vi "Terminate Session.vi"(8 "error in (no error)":errorcluster, 10 "Destroy (T)":bool=TRUE, 11 "Session in":refnum<class "Session.lvclass">) -> (0 "error out":errorcluster, 2 "Destroyed":bool, 3 "Session out":refnum<class "Session.lvclass">)   [LabVIEW 2013, in "MQTT Server.lvlib" / "Session.lvclass"]
doc: "Set the \"Destroy\" flag to True if the Connection Handler terminates to force the session to be destroyed for good, no matter what the CleanSession flag state is.\nIf the Connection Handler does not terminate and the CleanSession flag is false, then the Session's process stops but the last state of the session is maintained for a possible client reconnection."
uses:
  Session.lvclass
  Session.lvclass/Session.ctl
  Connection/TCPConnection.lvclass
  StoredSessions/StoredSessions.lvclass
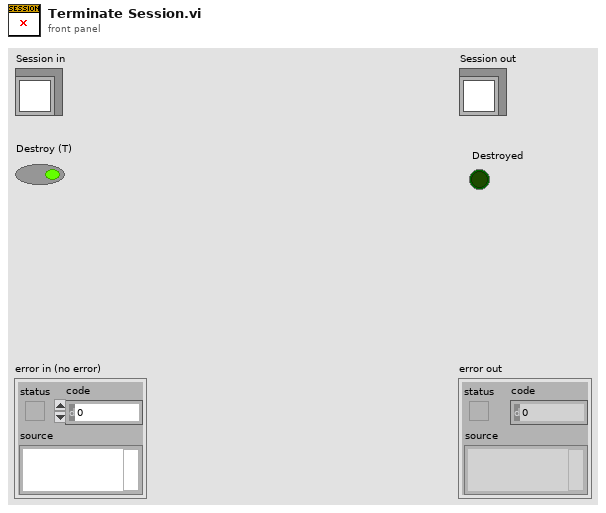
[diagram p1: front panel]
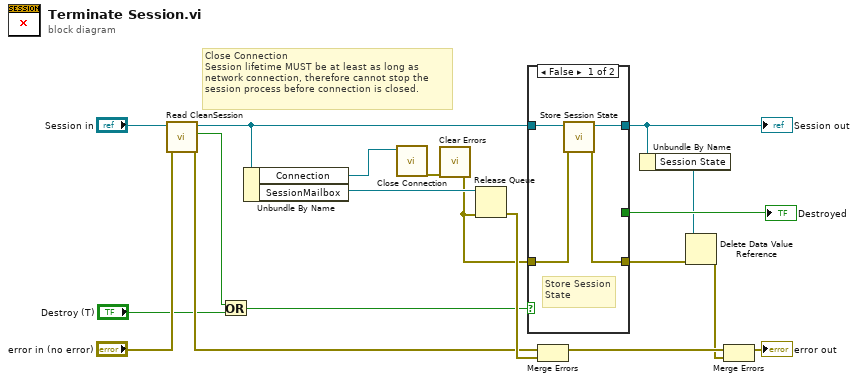
[diagram p0: block diagram]
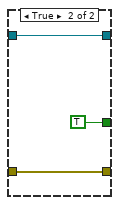
[diagram p2: hidden frame]
diagram:
  # "Close Connection\nSession lifetime MUST be at least as long as \nnetwork connection, therefore cannot stop the\nsession process before connection is closed."
  n1 = call "Read CleanSession.vi"("error in (no error)"="error in (no error)", "Session in"="Session in") -> ("error out"=w13:errorcluster, "CleanSession"=w1:bool, "Session out"=w4:refnum<class "Session.lvclass">)  [unwired: 7 in]
  n2 = Or(x=w1, y="Destroy (T)") -> (x .or. y?=w9:bool)
  n3 = Unbundle By Name(w4) -> ("Connection"=w16:refnum<class "TCPConnection.lvclass">, "SessionMailbox"=w17:refnum<queue>)
  n4 = call-dynamic "Close Connection.vi"("TCPConnection in"=w16) -> ("error out"=w15:errorcluster)  [unwired: 9 in, 1 out]
  n5 = call <vilib>:"Clear Errors.vi"("error in (no error)"=w15) -> ("error out"=w7:errorcluster)  [unwired: 6 in]
  n6 = Release Queue(queue=w17, error in (no error)=w7) -> (error out=w14:errorcluster)  [unwired: 1 in, 2 out]
  n7 = case shown="False" w9 {
    tunnel: [w22 w25] -> w5
    tunnel: [_ TRUE] -> w8
    tunnel: w7 -> [w23 w25]
    tunnel: [w20 w24] -> w3
    tunnel: w4 -> [w21 w24]
    frame False {
      # "Store Session\nState"
      n8 = call "Store Session State.vi"("error in (no error)"=w23, "Session"=w21) -> ("error out"=w22:errorcluster, "Session dup"=w20:refnum<class "Session.lvclass">)  [unwired: 8 in]
    }
    frame True {
    }
  }
  "Session out" <- w3
  "Destroyed" <- w8
  n9 = Merge Errors(w13, w14) -> (w11:errorcluster)
  n10 = Unbundle By Name(w3) -> ("Session State"=w2:refnum<data-value>)
  n11 = Delete Data Value Reference(data value reference=w2, error in=w5) -> (error out=w6:errorcluster)  [unwired: 1 out]
  n12 = Merge Errors(w11, w6) -> (→"error out":errorcluster)
